vi "Set_Sub_Collection.vi"(8 "error in (no error)":errorcluster caption="entrée d'erreur (pas d'erreur)", 11 "Firebase PCBA en entrée":refnum<class "Firebase Benches P2193.lvclass">) -> (0 "error out":errorcluster caption="sortie d'erreur", 3 "Firebase PCBA en sortie":refnum<class "Firebase Benches P2193.lvclass">)   [LabVIEW 2020, in "Library Instrument & Equipement.lvlib" / "Library FireBase.lvlib" / "Firebase Benches P2193.lvclass"]
doc: "Create New document\nPlease initialise the following values\n - Name BDD\n - Document of test sequence\n - API Key"
uses:
  Firebase Benches P2193.lvclass
  C:/Users/ngarcin/OneDrive - Altyor/Standard TB/Class/Firebase/Source/Firebase Driver/Firebase Driver.lvclass
  Firebase Benches P2193.lvclass/Firebase Benches P2193.ctl
  Firebase Altyor/Firebase Altyor.lvclass
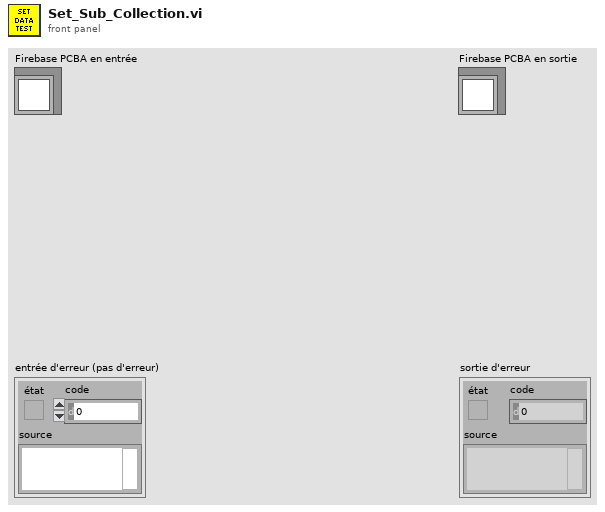
[diagram p1: front panel]
types:
  T1 = cluster{"Result":cluster{"booleanValue":bool}, "Name":cluster{"stringValue":string}, "StartOfTest":cluster{"timestampValue":string}, "EndOfTest":cluster{"timestampValue":string}, "limit":cluster{"mapValue":cluster{"fields":cluster{"Lower":cluster{"stringValue":string}, "Upper":cluster{"stringValue":string}}}}, "Value":cluster{"stringValue":string}, "Type":cluster{"stringValue":string}, "MainTest":cluster{"stringValue":string}}
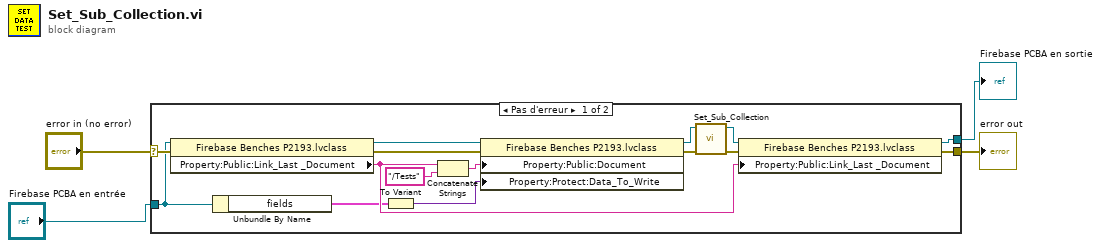
[diagram p0: block diagram]
diagram:
  n1 = case shown="Pas d'erreur" "error in (no error)" {
    selector: "error in (no error)" -> [w18 w21]
    tunnel: [w14 w21] -> w2
    tunnel: [w5 w20] -> w1
    tunnel: "Firebase PCBA en entrée" -> [w7 w20]
    frame No Error {
      n2 = property class="Firebase Benches P2193.lvclass"(reference=w7, error in=w18) -> (reference out=w17:refnum<class "Firebase Benches P2193.lvclass">, error out=w16:errorcluster, "Property:Public:Link_Last _Document"=w13:string)
      n3 = Unbundle By Name(w7) -> ("fields"=w6:T1)
      n4 = To Variant(anything=w6) -> (Variant=w12:variant)
      n5 = Concatenate Strings(w13, "/Tests" ("chaîne")) -> (w15:string)
      n6 = property class="Firebase Benches P2193.lvclass"(reference=w17, error in=w16, "Property:Public:Document"=w15, "Property:Protect:Data_To_Write"=w12) -> (reference out=w8:refnum<class "Firebase Benches P2193.lvclass">, error out=w11:errorcluster)
      n7 = call-parent "Set_Sub_Collection.vi"("error in (no error)"=w11, "Firebase PCBA en entrée"=w8) -> ("error out"=w10:errorcluster, "Firebase PCBA en sortie"=w9:refnum<class "Firebase Benches P2193.lvclass">)  [unwired: 8 in]
      n8 = property class="Firebase Benches P2193.lvclass"(reference=w9, error in=w10, "Property:Public:Link_Last _Document"=w13) -> (reference out=w5:refnum<class "Firebase Benches P2193.lvclass">, error out=w14:errorcluster)
    }
    frame Error {
    }
  }
  "error out" <- w2
  "Firebase PCBA en sortie" <- w1
